vi "VisaReadExample3.vi"() -> ()   [LabVIEW 2016]
uses:
  <vilib>/Instr/_visa.llb/VISA Configure Serial Port (Instr).vi
panel:
  out "size(s)":i32
  out "PULSE":string="126526"
  in  "Upper Cut-Off":dbl=100.0
  in  "Lower Cut-Off":dbl=10.0
  in  "OK Button":bool
  out "Waveform Graph":dynamicdata(graph)
  in  "Array 2":dbl[](array[numeric])=array[6515 elements]
  in  "Array":dbl[](array[numeric])=array[6516 elements]
  out "substring 2":string="I"
  out "substring":string="126526"
  out "read buffer":string="I126526"
  in  "VISA resource name":refnum<visa-resource-name>="COM3"
  in  "stop":bool
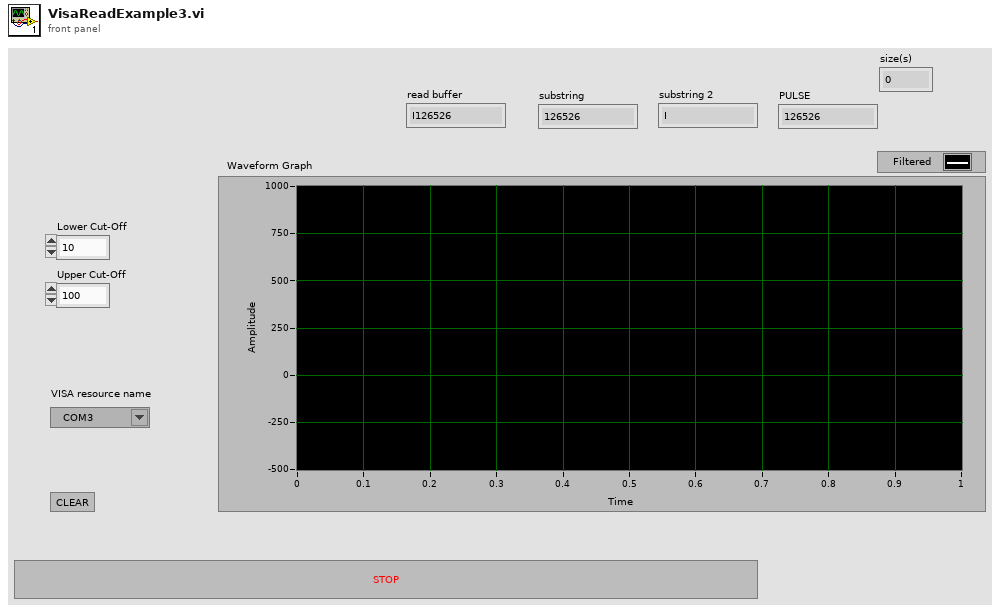
[diagram p1: front panel]
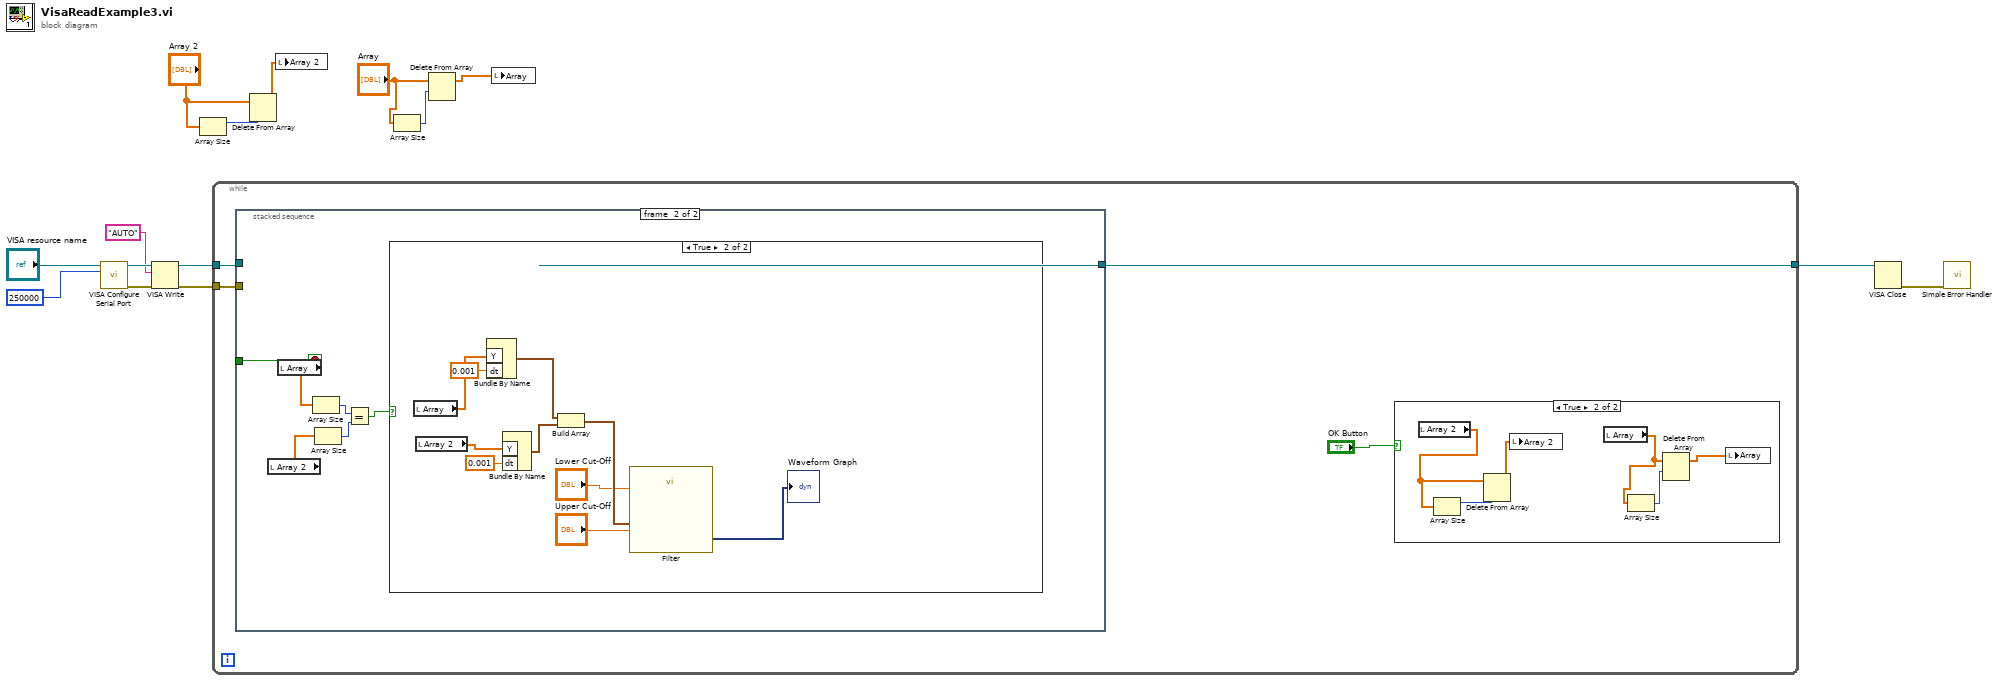
[diagram p0: block diagram]
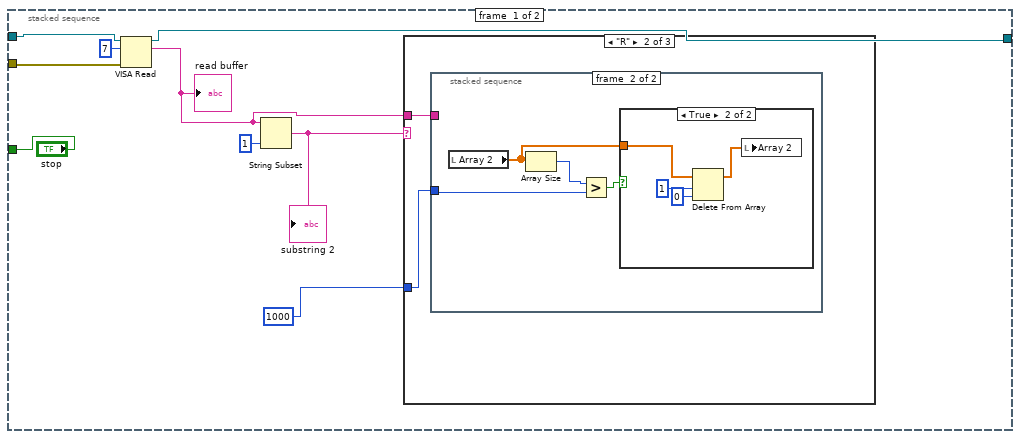
[diagram p3: hidden frame]
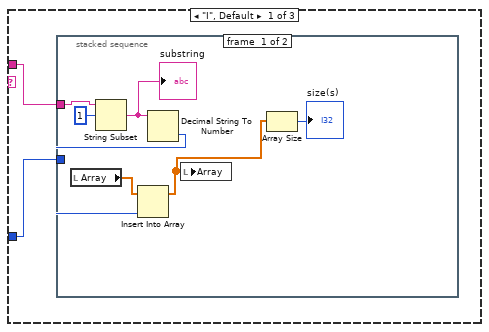
[diagram p4: hidden frame]
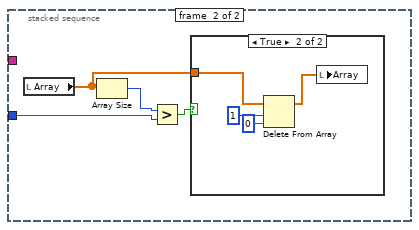
[diagram p5: hidden frame]
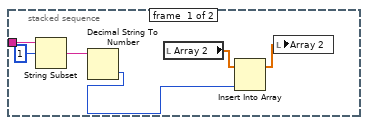
[diagram p7: hidden frame]
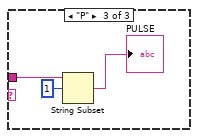
[diagram p9: hidden frame]
diagram:
  n1 = call-poly "VISA Configure Serial Port"("VISA resource name"="VISA resource name", "baud rate (9600)"=u32 250000) -> ("VISA resource name out"=w11:refnum<visa-resource-name>, "error out"=w9:errorcluster)  [unwired: 12 in]
  n2 = VISA Write(VISA resource name=w11, write buffer="AUTO", error in (no error)=w9) -> (VISA resource name out=w10:refnum<visa-resource-name>, error out=w8:errorcluster)  [unwired: 1 out]
  n3 = Array Size(array="Array 2") -> (size(s)=w3:i32)
  n4 = while {
    tunnel: [w19] -> w14
    tunnel: w10 -> [w18]
    tunnel: w8 -> [w17]
    stop <- w20 stop-if-true
    n5 = stacked-sequence {
      tunnel: ["stop" _] -> w20
      tunnel: [w34 _] -> w19
      tunnel: w18 -> [w32 _]
      tunnel: w17 -> [w29 _]
      frame #0 {
        n6 = VISA Read(VISA resource name=w32, byte count=u32 7, error in (no error)=w29) -> (VISA resource name out=w34:refnum<visa-resource-name>, read buffer=w28:string)  [unwired: 2 out]
        "read buffer" <- w28
        n7 = String Subset(string=w28, length (rest)=1 ("length (rest)")) -> (substring=w30:string)  [unwired: 1 in]
        "substring 2" <- w30
        n8 = case shown="\"R\"" w30 {
          tunnel: w28 -> [w37 w54 w69]
          tunnel: 1000 ("y") -> [w36 w53 _]
          frame "I", Default {
            n9 = stacked-sequence {
              tunnel: w37 -> [w43 _]
              tunnel: w36 -> [_ w47]
              frame #0 {
                n10 = local read "Array"() -> (w41:dbl[])
                n11 = String Subset(string=w43, offset (0)=1) -> (substring=w42:string)  [unwired: 1 in]
                "substring" <- w42
                n12 = Decimal String To Number(string=w42) -> (number=w40:i32)  [unwired: 2 in, 1 out]
                n13 = Insert Into Array(array=w41, new element=w40) -> (w39:dbl[])  [unwired: 1 in]
                n14 = local write "Array"(w39) -> ()
                n15 = Array Size(array=w39) -> (size(s)=→"size(s)":i32)
              }
              frame #1 {
                n16 = local read "Array"() -> (w45:dbl[])
                n17 = Array Size(array=w45) -> (size(s)=w48:i32)
                n18 = Greater?(x=w48, y=w47) -> (0:w46:bool)
                n19 = case shown="True" w46 {
                  tunnel: w45 -> [_ w52]
                  frame False {
                  }
                  frame True {
                    n20 = Delete From Array(array=w52, length=1, index=0) -> (array with subset deleted=w49:dbl[])  [unwired: 1 out]
                    n21 = local write "Array"(w49) -> ()
                  }
                }
              }
            }
          }
          frame "R" {
            n22 = stacked-sequence {
              tunnel: w54 -> [w60 _]
              tunnel: w53 -> [_ w61]
              frame #0 {
                n23 = String Subset(string=w60, offset (0)=1) -> (substring=w58:string)  [unwired: 1 in]
                n24 = Decimal String To Number(string=w58) -> (number=w56:i32)  [unwired: 2 in, 1 out]
                n25 = local read "Array 2"() -> (w57:dbl[])
                n26 = Insert Into Array(array=w57, new element=w56) -> (w55:dbl[])  [unwired: 1 in]
                n27 = local write "Array 2"(w55) -> ()
              }
              frame #1 {
                n28 = local read "Array 2"() -> (w62:dbl[])
                n29 = Array Size(array=w62) -> (size(s)=w64:i32)
                n30 = Greater?(x=w64, y=w61) -> (0:w63:bool)
                n31 = case shown="True" w63 {
                  tunnel: w62 -> [_ w68]
                  frame False {
                  }
                  frame True {
                    n32 = Delete From Array(array=w68, length=1, index=0) -> (array with subset deleted=w65:dbl[])  [unwired: 1 out]
                    n33 = local write "Array 2"(w65) -> ()
                  }
                }
              }
            }
          }
          frame "P" {
            n34 = String Subset(string=w69, offset (0)=1) -> (substring=→"PULSE":string)  [unwired: 1 in]
          }
        }
      }
      frame #1 {
        n35 = local read "Array 2"() -> (w76:dbl[])
        n36 = local read "Array"() -> (w75:dbl[])
        n37 = Array Size(array=w75) -> (size(s)=w74:i32)
        n38 = Array Size(array=w76) -> (size(s)=w73:i32)
        n39 = Equal?(x=w74, y=w73) -> (x = y?=w72:bool)
        n40 = case shown="True" w72 {
          frame False {
          }
          frame True {
            n41 = local read "Array"() -> (w86:dbl[])
            n42 = local read "Array 2"() -> (w85:dbl[])
            n43 = Bundle By Name("Y"=w86, "dt"=0.001) -> (w81:waveform(dbl))  [unwired: 1 in]
            n44 = Bundle By Name("Y"=w85, "dt"=0.001) -> (w82:waveform(dbl))  [unwired: 1 in]
            n45 = Build Array(w81, w82) -> (w80:waveform(dbl)[])
            n46 = call "Filter"("Lower Cut-Off"="Lower Cut-Off", "Upper Cut-Off"="Upper Cut-Off", "Signal"=w80) -> ("Filtered Signal"=→"Waveform Graph":dynamicdata)  [unwired: 7 in, 1 out]
          }
        }
      }
    }
    n47 = case shown="True" "OK Button" {
      frame False {
      }
      frame True {
        n48 = local read "Array 2"() -> (w22:dbl[])
        n49 = Array Size(array=w22) -> (size(s)=w25:i32)
        n50 = Delete From Array(array=w22, length=w25) -> (array with subset deleted=w24:dbl[])  [unwired: 1 in, 1 out]
        n51 = local write "Array 2"(w24) -> ()
        n52 = local read "Array"() -> (w21:dbl[])
        n53 = Array Size(array=w21) -> (size(s)=w26:i32)
        n54 = Delete From Array(array=w21, length=w26) -> (array with subset deleted=w23:dbl[])  [unwired: 1 in, 1 out]
        n55 = local write "Array"(w23) -> ()
      }
    }
  }
  n56 = Delete From Array(array="Array 2", length=w3) -> (array with subset deleted=w5:dbl[])  [unwired: 1 in, 1 out]
  n57 = local write "Array 2"(w5) -> ()
  n58 = Array Size(array="Array") -> (size(s)=w1:i32)
  n59 = Delete From Array(array="Array", length=w1) -> (array with subset deleted=w6:dbl[])  [unwired: 1 in, 1 out]
  n60 = local write "Array"(w6) -> ()
  n61 = VISA Close(VISA resource name=w14) -> (error out=w13:errorcluster)  [unwired: 1 in]
  n62 = call <vilib>:"Simple Error Handler.vi"("error in (no error)"=w13) -> ()  [unwired: 4 in, 5 out]
